vi "RSZVB Send Trigger and Wait for OPC.vi"(8 "error in (no error)":errorcluster {"code" format="%.0x"}, 10 "Timeout (15000)":i32=15000, 11 "VISA session":refnum<visa-resource-name>) -> (0 "error out":errorcluster {"code" format="%.0x"}, 3 "dup VISA session":refnum<visa-resource-name>)   [LabVIEW 2011]
doc: "This VI triggers all actions waiting for a trigger event in the selected window and waits for operation completed (OPC) before returning the status code.\n\nRemote-control command(s):\n*TRG\n*OPC?"
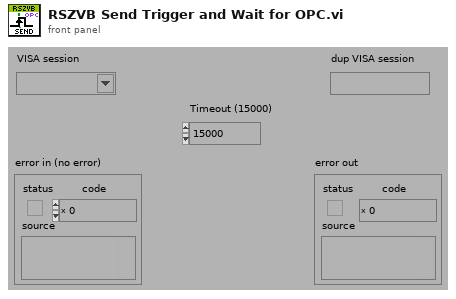
[diagram p1: front panel]
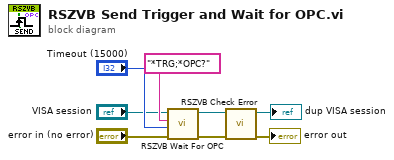
[diagram p0: block diagram]
diagram:
  n1 = call "RSZVB Wait For OPC.vi"("error in (no error)"="error in (no error)", "Timeout (300000 ms)"="Timeout (15000)", "Command"="*TRG;*OPC?", "VISA session"="VISA session") -> ("error out"=w8:errorcluster, "dup VISA session"=w7:refnum<visa-resource-name>)  [unwired: 5 in, 1 out]
  n2 = call "RSZVB Check Error.vi"("error in (no error)"=w8, "VISA session"=w7) -> ("error out"=→"error out":errorcluster, "dup VISA session"=→"dup VISA session":refnum<visa-resource-name>)  [unwired: 8 in]
